vi "GetStrBe.vi"(3 "error in":errorcluster caption="错误输入", 4 "nchars":i32, 5 "refnum in":refnum<file>) -> (0 "error out":errorcluster, 1 "str":string, 2 "refnum out":refnum<file>)   [LabVIEW 2016]
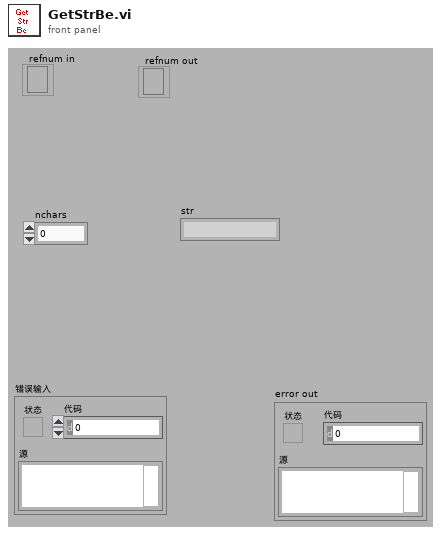
[diagram p1: front panel]
types:
  T1 = enum16{"big-endian, network order", "native, host order", "little-endian"}
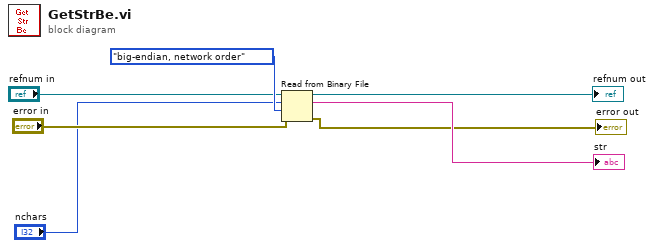
[diagram p0: block diagram]
diagram:
  n1 = Read from Binary File(8:"error in", 9:T1."big-endian, network order" ("字节顺序(0:big-endian, network order)"), 10:"nchars", 11:"refnum in") -> (0:→"error out":errorcluster, 2:→"str":string, 3:→"refnum out":refnum<file>)  [unwired: 3 out]
